vi "Restore Default Symbols.vi"(8 "错误输入":errorcluster, 11 "Listbox Ref":refnum<vi>) -> (0 "错误输出":errorcluster, 3 "Dup Listbox Ref":refnum<vi>)   [LabVIEW 2011, in "Listbox Tool.lvlib"]
uses:
  Listbox Tool.lvlib
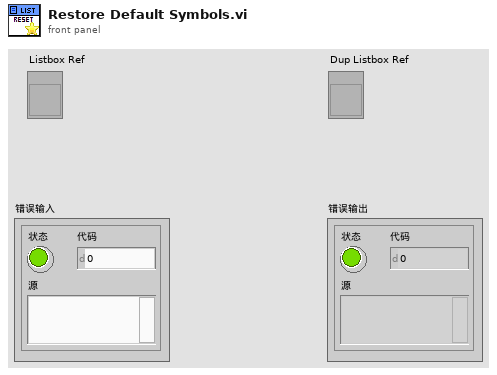
[diagram p1: front panel]
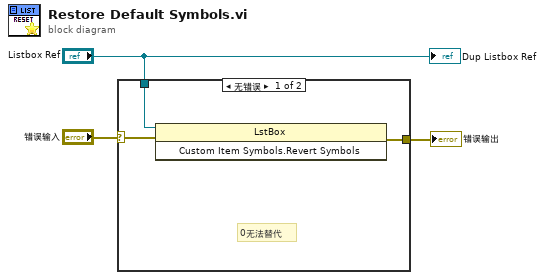
[diagram p0: block diagram]
diagram:
  n1 = case shown="无错误" "错误输入" {
    selector: "错误输入" -> [w5 w7]
    tunnel: [w4 w7] -> w2
    tunnel: "Listbox Ref" -> [w6 _]
    frame No Error {
      # "0无法替代"
      n2 = invoke class="LstBox" method="Custom Item Symbols.Revert Symbols"(reference=w6, error in=w5) -> (error out=w4:errorcluster)  [unwired: 1 in, 2 out]
    }
    frame Error {
    }
  }
  "错误输出" <- w2
  "Dup Listbox Ref" <- "Listbox Ref"
